vi "Shutdown Logger.vi"(8 "error in":errorcluster, 9 "timeout in ms (5000)":i32=5000, 11 "Log Producer in":T1) -> (0 "error out":errorcluster, 3 "Log Producer out":T1)   [LabVIEW 2020, in "Frame Logging.lvlib"]
uses:
  Frame Logging.lvlib
  Log_Producer.ctl
  Message_Request.ctl
  Message_Request_Action.ctl
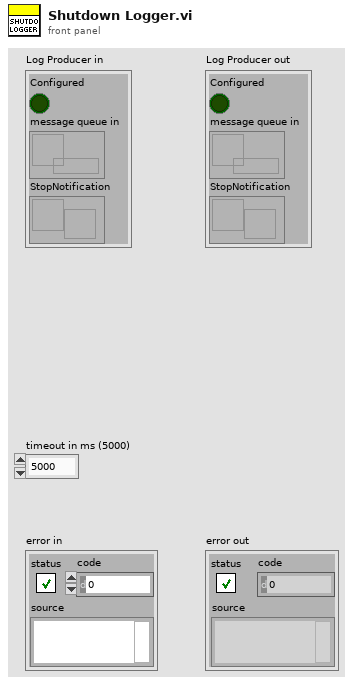
[diagram p1: front panel]
types:
  T1 = typedef "Frame Logging.lvlib/Log_Producer.ctl" = cluster{"Configured":bool, "message queue in":refnum<queue>, "StopNotification":refnum<notifier>}
  T2 = typedef "Frame Logging.lvlib/Message_Request_Action.ctl" = enum16{"Initialize", "Open File", "Log", "Manage Disk", "Stop", "Close File", "Update Configuration"}
  T3 = typedef "Frame Logging.lvlib/Message_Request.ctl" = cluster{"request":T2, "data":variant}
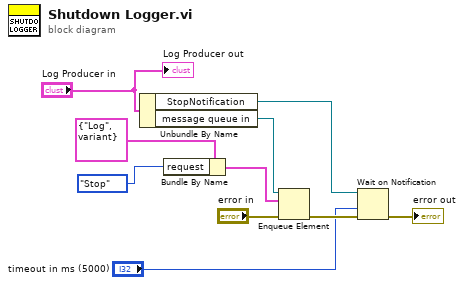
[diagram p0: block diagram]
diagram:
  n1 = Unbundle By Name("Log Producer in") -> ("StopNotification"=w4:refnum<notifier>, "message queue in"=w9:refnum<queue>)
  n2 = Bundle By Name(cluster=T3 {"request"=enum."Log", "data"=variant} ("Message_type"), "request"=Message_Request_Action."Stop") -> (w8:T3)
  n3 = Enqueue Element(queue=w9, element=w8, error in (no error)="error in") -> (error out=w3:errorcluster)  [unwired: 1 in, 2 out]
  n4 = Wait on Notification(notifier=w4, timeout in ms (-1)="timeout in ms (5000)", error in (no error)=w3) -> (error out=→"error out":errorcluster)  [unwired: 1 in, 3 out]
  "Log Producer out" <- "Log Producer in"
